vi "UDP Receive (core).vi"(7 "timeout ms (100)":i32=100, 8 "error in (no error)":errorcluster, 9 "eSCL Cmd (send)":string="PR", 11 "connection ID in":refnum<k16>) -> (0 "error out":errorcluster, 1 "Received Data":T1, 2 "ACK/NACK":T2, 3 "connection ID out":refnum<k16>)   [LabVIEW 2016, in "SMD-7615.lvlib" / "eSCL.lvlib"]
uses:
  eSCL.lvlib
  UDP ACK NACK.ctl
  UDP Received Data.ctl
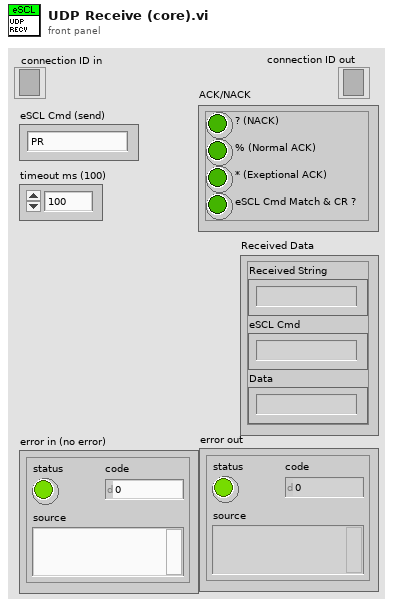
[diagram p1: front panel]
types:
  T1 = typedef "SMD-7615.lvlib/eSCL.lvlib/UDP Received Data.ctl" = cluster{"Received String":string, "eSCL Cmd":string, "Data":string}
  T2 = typedef "SMD-7615.lvlib/eSCL.lvlib/UDP ACK NACK.ctl" = cluster{"? (NACK)":bool, "% (Normal ACK)":bool, "* (Exeptional ACK)":bool, "eSCL Cmd Match & CR ?":bool}
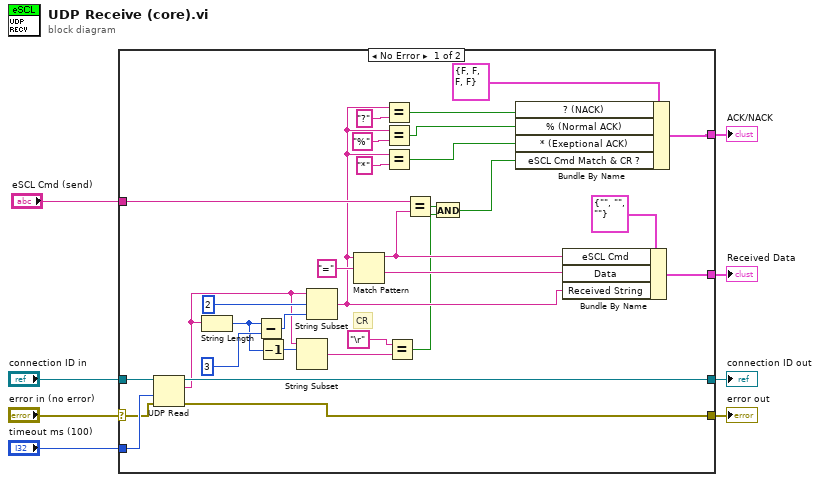
[diagram p0: block diagram]
diagram:
  n1 = case shown="No Error" "error in (no error)" {
    selector: "error in (no error)" -> [w38 w40]
    tunnel: "connection ID in" -> [w31 w41]
    tunnel: [w36 w41] -> w6
    tunnel: [w37 w40] -> w5
    tunnel: "timeout ms (100)" -> [w39 _]
    tunnel: [w23 _] -> w3
    tunnel: "eSCL Cmd (send)" -> [w22 _]
    tunnel: [w18 _] -> w1
    frame No Error {
      # "CR"
      n2 = UDP Read(connection ID=w31, timeout ms (25000)=w39, 8:w38) -> (data out=w16:string, error out=w37:errorcluster, 3:w36:refnum<k16>)  [unwired: 1 in, 2 out]
      n3 = String Length(string=w16) -> (length=w14:i32)
      n4 = Subtract(x=w14, y=3) -> (x-y=w33:i32)
      n5 = Decrement(x=w14) -> (x-1=w15:i32)
      n6 = String Subset(string=w16, offset (0)=w15) -> (substring=w13:string)  [unwired: 1 in]
      n7 = String Subset(string=w16, offset (0)=2, length (rest)=w33) -> (substring=w17:string)
      n8 = Match Pattern(string=w17, regular expression="=") -> (before substring=w20:string, after substring=w19:string)  [unwired: 1 in, 2 out]
      n9 = Equal?(x=w17, y="?") -> (x = y?=w26:bool)
      n10 = Equal?(x=w17, y="%") -> (x = y?=w25:bool)
      n11 = Equal?(x=w17, y="*") -> (x = y?=w24:bool)
      n12 = Equal?(x="\r", y=w13) -> (x = y?=w9:bool)
      n13 = Equal?(x=w22, y=w20) -> (x = y?=w11:bool)
      n14 = And(x=w11, y=w9) -> (x .and. y?=w10:bool)
      n15 = Bundle By Name(cluster=T2 {"? (NACK)"=FALSE, "% (Normal ACK)"=FALSE, "* (Exeptional ACK)"=FALSE, "eSCL Cmd Match & CR ?"=FALSE} ("ACK/NACK 2"), "? (NACK)"=w26, "% (Normal ACK)"=w25, "* (Exeptional ACK)"=w24, "eSCL Cmd Match & CR ?"=w10) -> (w23:T2)
      n16 = Bundle By Name(cluster=T1 {"Received String"="", "eSCL Cmd"="", "Data"=""} ("Received Data 2"), "eSCL Cmd"=w20, "Data"=w19, "Received String"=w17) -> (w18:T1)
    }
    frame Error {
    }
  }
  "connection ID out" <- w6
  "error out" <- w5
  "ACK/NACK" <- w3
  "Received Data" <- w1
